vi "Waveform Settings Write.vi"(4 "error in (no error)":errorcluster, 5 "Value":T3={"Type"=enum."Sine", "Periods"=0.0, "Points"=0, "Offset"=0.0, "Amplitdue"=0.0, "Phase"=0.0, "func"=""}, 6 "Container State":T2, 7 "Display State In":T1) -> (0 "error out":errorcluster, 3 "Display State Out":T1)   [LabVIEW 2012, in "Waveform Control.xctl"]
uses:
  Waveform Control.xctl
  <vilib>/_xctls/Container State.ctl
  subvis/FP Controls.ctl
  subvis/Function Types.ctl
  Controls/State.ctl
  Controls/Volatile State Ops.ctl
  <vilib>/_xctls/XControlSupport.lvlib
panel:
  # "Replace the Value Control below with a Control of desired type.\nDo not remove this Control or the others from the connector pane.\nDo not change the connector pane pattern.\nThe Value control should always be the third terminal from top on the input side in the connector pane."
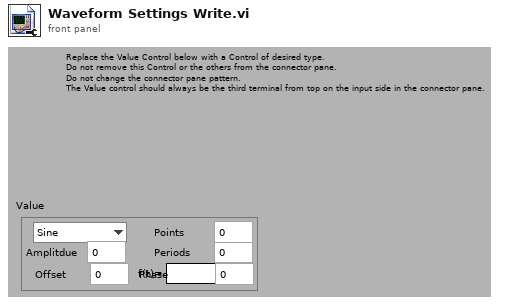
[diagram p1: front panel]
types:
  T1 = typedef "Waveform Control.xctl/State.ctl" = cluster{"Name":string}
  T2 = typedef "XControlSupport.lvlib/Container State.ctl" = cluster{"Indicator?":bool, "Run Mode?":bool, " Refnum":refnum<vi>}
  T3 = typedef "Waveform Control.xctl/FP Controls.ctl" = cluster{"Type":T4, "Periods":dbl, "Points":i32, "Offset":dbl, "Amplitdue":dbl, "Phase":dbl, "func":string}
  T4 = typedef "Waveform Control.xctl/Function Types.ctl" = enum16{"Level", "Sine", "Triangle", "Ramp", "Saw Tooth", "Square", "Function"}
  T5 = typedef "Waveform Control.xctl/Volatile State Ops.ctl" = enum16{"Read", "Write", "Update State from Data"}
  T6 = typedef "Waveform Control.xctl/Waveform State.ctl" = cluster{"Show Axes":bool, "Show Y=0":bool, "Controls":T3, "Show Current Location":bool, "Current Location":i32, "dt":dbl, "t0":timestamp, "Format and Units":string}
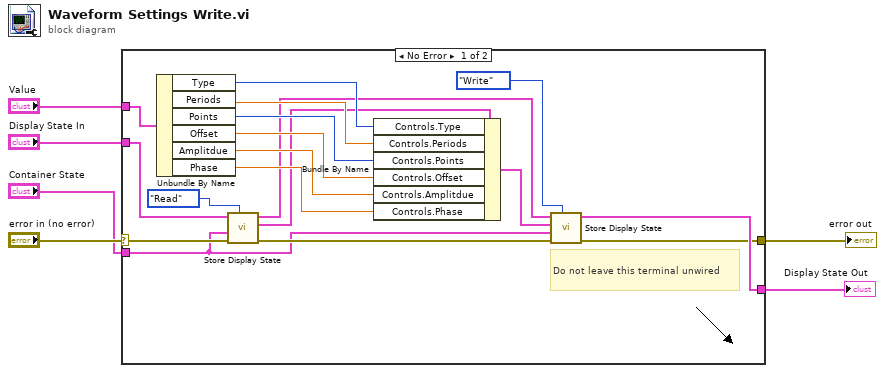
[diagram p0: block diagram]
diagram:
  n1 = case shown="No Error" "error in (no error)" {
    selector: "error in (no error)" -> [w10 w25]
    tunnel: "Display State In" -> [w18 w26]
    tunnel: [w8 w25] -> w5
    tunnel: [w13 w26] -> w4
    tunnel: "Value" -> [w9 _]
    tunnel: "Container State" -> [w7 _]
    frame No Error {
      # "Do not leave this terminal unwired"
      n2 = Unbundle By Name(w9) -> ("Type"=w24:T4, "Periods"=w23:dbl, "Points"=w22:i32, "Offset"=w21:dbl, "Amplitdue"=w20:dbl, "Phase"=w19:dbl)
      n3 = call "Store Display State.vi"("Operation In"=Volatile_State_Ops."Read" ("Operation"), "Error In (no Error) In"=w10, "Container State In"=w7, "State In"=w18) -> ("Error Out"=w16:errorcluster, "Waveform State Out"=w17:T6, "Display State Out"=w14:T1)  [unwired: 2 in, 3 out]
      n4 = Bundle By Name(cluster=w17, "Controls.Type"=w24, "Controls.Periods"=w23, "Controls.Points"=w22, "Controls.Offset"=w21, "Controls.Amplitdue"=w20, "Controls.Phase"=w19) -> (w15:T6)
      n5 = call "Store Display State.vi"("Operation In"=Volatile_State_Ops."Write" ("Operation"), "Error In (no Error) In"=w16, "Container State In"=w7, "Waveform State In"=w15, "State In"=w14) -> ("Error Out"=w8:errorcluster, "Display State Out"=w13:T1)  [unwired: 1 in, 4 out]
    }
    frame Error {
    }
  }
  "error out" <- w5
  "Display State Out" <- w4
